vi "sub_bonding-force2.vi"(8 "error in":errorcluster caption="에러 입력(에러 없음)", 11 "wf sum in":waveform(dbl) caption="sum of wf") -> (0 "error out":errorcluster caption="에러 출력")   [LabVIEW 2013]
uses:
  <vilib>/measure/mamon.llb/Trigger Detection for 1 Channel.vi
  <vilib>/Waveform/WDTOps.llb/WDT Get Waveform Subset DBL.vi
  <vilib>/measure/mascope.llb/Amplitude and Levels 1 chan.vi
  <vilib>/measure/NI_MAPro.lvlib
panel:
  out "dt":dbl
  out "amplitude":dbl caption="진폭" format="%.2p"
  out "웨이브폼 그래프 2":waveform(dbl)(graph)
  out "웨이브폼 그래프":waveform(dbl)(graph)
  out "Y max":dbl caption="Y 최대" format="%0.2f"
  out "Y min":dbl caption="Y 최소" format="%0.2f"
  out "high state level":dbl caption="높은 상태 레벨" format="%.2g"
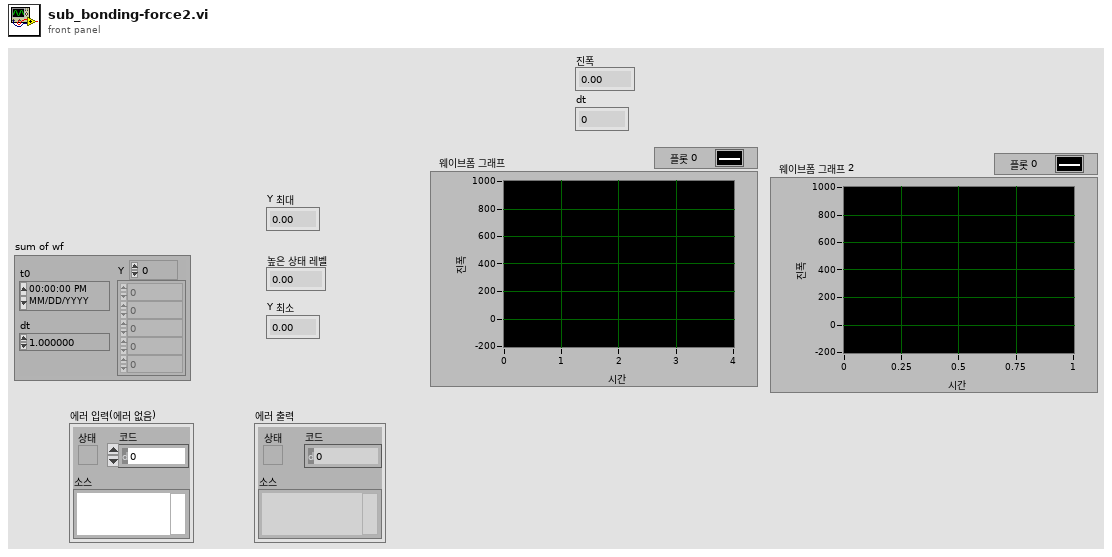
[diagram p1: front panel]
types:
  T1 = typedef "config_ctl.ctl" = cluster{"Trigger minlevel":dbl, "Lower Cut-Off":dbl, "Force high_level":dbl, "state settings":cluster{"method":enum32{"histogram", "peak", "auto select"}, "histogram size":i32, "histogram method":enum16{"mode"}, "reserved":dbl}, "SPA-300 Setting":cluster{"Bonding force (g)":dbl, "Bonding time (ms)":dbl, "Pickup force (g)":dbl, "Pickup time (ms)":dbl, "Speed":enum16{"Slow", "Fast"}}}
  T2 = typedef "UI_ctl.ctl" = cluster{"vacuum 차트":refnum<vi>, "vacuum":refnum<vi>, "Strain raw graph":refnum<vi>, "Strain raw chart":refnum<vi>, "Bonding time":refnum<vi>, "Bonding force":refnum<vi>, "Balance":refnum<vi>, "Filtered force graph":refnum<vi>, "ROI intensity":refnum<vi>, "Heater_rt":refnum<vi>, "Tensile force":refnum<vi>}
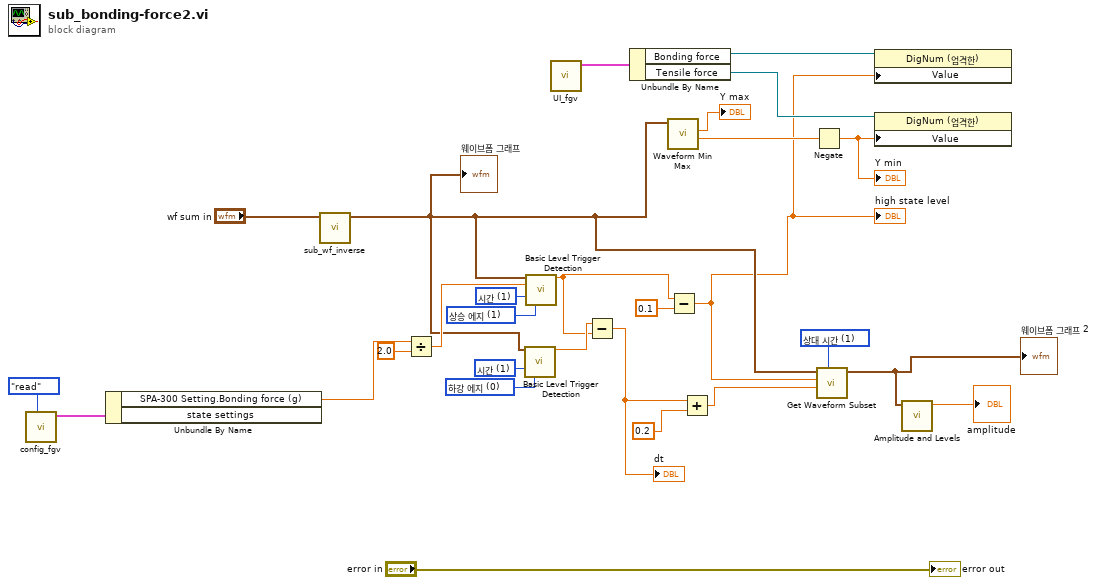
[diagram p0: block diagram]
diagram:
  w9 = u16 1 items=["샘플 ", "상대 시간"] ("start/duration format")
  w14 = u16 0 items=["하강 에지", "상승 에지"] ("trigger slope")
  w15 = u16 1 items=["인덱스", "시간"] ("location mode")
  w16 = u16 1 items=["하강 에지", "상승 에지"] ("trigger slope")
  w17 = u16 1 items=["인덱스", "시간"] ("location mode")
  n1 = call "config_fgv.vi"("cmd"=enum16{"write", "read", "ini"}."read") -> ("Config out"=w26:T1)  [unwired: 9 in, 1 out]
  n2 = Unbundle By Name(w26) -> ("SPA-300 Setting.Bonding force (g)"=w20:dbl)  [unwired: 1 out]
  n3 = call "sub_wf_inverse.vi"("Trigger graph"="wf sum in") -> ("inverse graph"=w10:waveform(dbl))  [unwired: 10 in]
  "웨이브폼 그래프" <- w10
  n4 = Divide(x=w20, y=2.0) -> (x/y=w18:dbl)
  n5 = call-poly <vilib>:"Basic Level Trigger Detection.vi"("signal in"=w10, "location mode"=w15, "trigger slope"=w14) -> ("trigger location"=w12:dbl)  [unwired: 10 in, 2 out]
  n6 = call-poly <vilib>:"Basic Level Trigger Detection.vi"("signal in"=w10, "level"=w18, "location mode"=w17, "trigger slope"=w16) -> ("trigger location"=w8:dbl)  [unwired: 9 in, 2 out]
  n7 = call "UI_fgv.vi"() -> ("UI cluster out"=w27:T2)  [unwired: 11 in]
  n8 = Subtract(x=w12, y=w8) -> (x-y=w6:dbl)
  "dt" <- w6
  n9 = Unbundle By Name(w27) -> ("Bonding force"=w28:refnum<vi>, "Tensile force"=w24:refnum<vi>)
  n10 = call <vilib>:"Waveform Min Max.vi"("waveform in"=w10) -> ("Y min"=w23:dbl, "Y max"=→"Y max":dbl)  [unwired: 5 in, 4 out]
  n11 = Subtract(x=w8, y=0.1) -> (x-y=w7:dbl)
  "high state level" <- w7
  n12 = Add(x=w6, y=0.2) -> (x+y=w4:dbl)
  n13 = Negate(x=w23) -> (-x=w22:dbl)
  "Y min" <- w22
  n14 = call-poly <vilib>:"Get Waveform Subset.vi"("start/duration format"=w9, "duration"=w4, "start samples/time"=w7, "waveform in"=w10) -> ("waveform out"=w1:waveform(dbl))  [unwired: 2 in, 3 out]
  "웨이브폼 그래프 2" <- w1
  n15 = property class="DigNum (엄격한)"(reference=w28, "Value"=w7) -> ()  [unwired: 1 in, 2 out]
  n16 = property class="DigNum (엄격한)"(reference=w24, "Value"=w22) -> ()  [unwired: 1 in, 2 out]
  n17 = call-poly <vilib>:"Amplitude and Levels.vi"("signal in"=w1) -> ("amplitude"=→"amplitude":dbl)  [unwired: 7 in, 3 out]
  "error out" <- "error in"
